vi "Read All Voltages.vi"(8 "error in (no error)":errorcluster, 11 "Analog-Output in":refnum<class "Analog-Output.lvclass">) -> (0 "error out":errorcluster, 2 "Voltages":dbl[](array[numeric]), 3 "Analog-Output out":refnum<class "Analog-Output.lvclass">)   [LabVIEW 2019, in "Analog-Output.lvlib" / "Analog-Output.lvclass"]
uses:
  Library/Analog-Output.lvclass
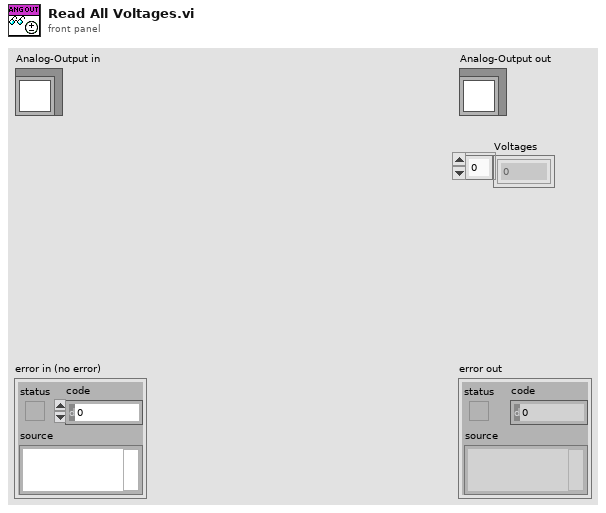
[diagram p1: front panel]
types:
  T1 = typedef "Analog-Output.lvlib/Analog-Output.lvclass/Settings.ctl" = cluster{"Voltage":dbl}
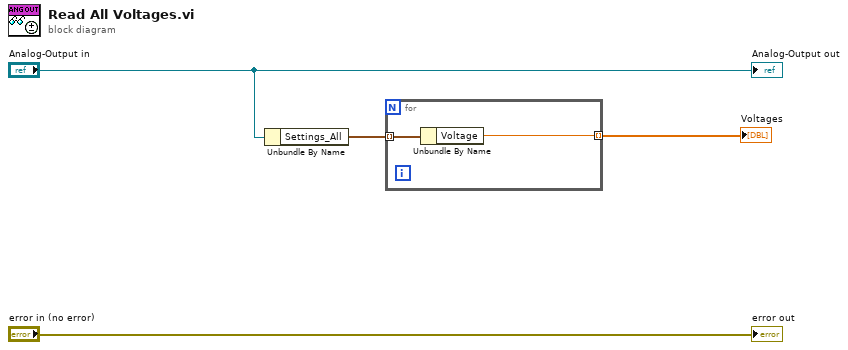
[diagram p0: block diagram]
diagram:
  n1 = Unbundle By Name("Analog-Output in") -> ("Settings_All"=w1:T1[])
  n2 = for {
    tunnel: w1 -> [w6] mode=indexing
    tunnel: [w5] -> w2 mode=indexing
    n3 = Unbundle By Name(w6) -> ("Voltage"=w5:dbl)
  }
  "Voltages" <- w2
  "error out" <- "error in (no error)"
  "Analog-Output out" <- "Analog-Output in"
